vi "Read RFSG Session.vi"(8 "error in (no error)":errorcluster, 11 "Scalar Path in":refnum<class "Scalar Path.lvclass">) -> (0 "error out":errorcluster, 2 "RFSG Session":refnum<k15>, 3 "Scalar Path out":refnum<class "Scalar Path.lvclass">)   [LabVIEW 2023, in "RFFixtureCharact.Public.lvlib" / "Scalar Path.lvclass"]
uses:
  Scalar Path.lvclass
  Scalar Path.lvclass/Scalar Path.ctl
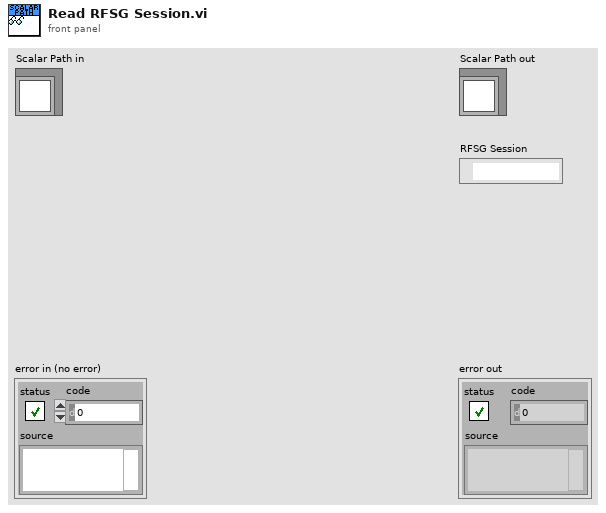
[diagram p1: front panel]
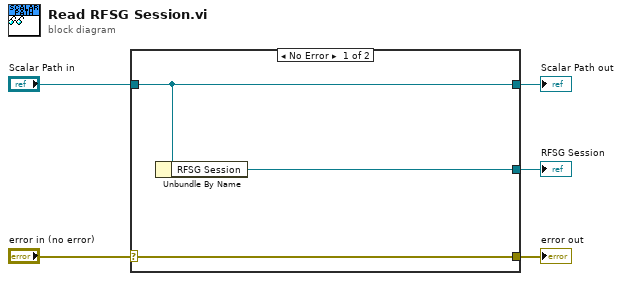
[diagram p0: block diagram]
diagram:
  n1 = case shown="No Error" "error in (no error)" {
    selector: "error in (no error)" -> [w8 w9]
    tunnel: [w8 w9] -> w4
    tunnel: [w7 w10] -> w2
    tunnel: "Scalar Path in" -> [w7 w10]
    tunnel: [w6 _] -> w1
    frame No Error {
      n2 = Unbundle By Name(w7) -> ("RFSG Session"=w6:refnum<k15>)
    }
    frame Error {
    }
  }
  "error out" <- w4
  "Scalar Path out" <- w2
  "RFSG Session" <- w1
